vi "PathPlanner_BoolCmdSamplingFilter.vi"(8 "Pecentage of Passing":dbl=0.1 format="%#_13g", 9 "Samples":i32=20, 11 "Input":bool) -> (3 "Output":bool)   [LabVIEW 2023]
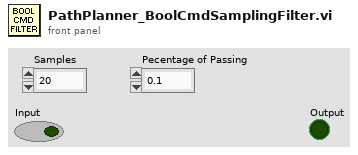
[diagram p1: front panel]
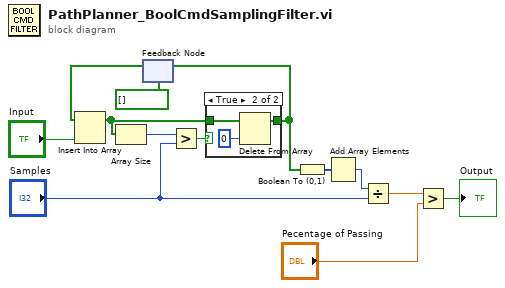
[diagram p0: block diagram]
diagram:
  n1 = feedback #1(bool[] []) -> (w9:bool[])
  n2 = Insert Into Array(array=w9, new element="Input") -> (w11:bool[])  [unwired: 1 in]
  n3 = Array Size(array=w11) -> (size(s)=w12:i32)
  n4 = Greater?(x=w12, y="Samples") -> (0:w13:bool)
  n5 = case shown="True" w13 {
    tunnel: w11 -> [w14 w17]
    tunnel: [w14 w16] -> w7
    frame False {
    }
    frame True {
      n6 = Delete From Array(array=w17, index=0) -> (array with subset deleted=w16:bool[])  [unwired: 1 in, 1 out]
    }
  }
  n7 = feedback-in #1(w7) -> ()
  n8 = Boolean To (0,1)(Boolean=w7) -> (0, 1=w6:i16[])
  n9 = Add Array Elements(numeric array=w6) -> (sum=w5:i16)
  n10 = Divide(x=w5, y="Samples") -> (x/y=w3:dbl)
  n11 = Greater?(x=w3, y="Pecentage of Passing") -> (0:→"Output":bool)
